vi "SetWaveLineColor.vi"(10 "曲线条数":u8, 11 "WaveformGraph输入":refnum<vi>) -> ()   [LabVIEW 2012, in "WaveGraphX.xctl"]
uses:
  WaveGraphX.xctl
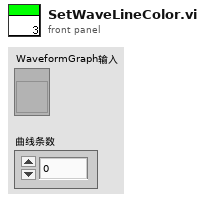
[diagram p1: front panel]
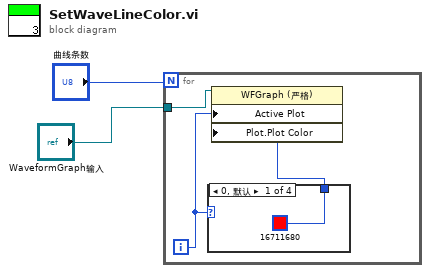
[diagram p0: block diagram]
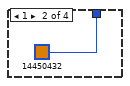
[diagram p2: hidden frame]
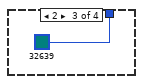
[diagram p3: hidden frame]
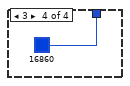
[diagram p4: hidden frame]
diagram:
  n1 = for {
    N: "曲线条数" -> [_]
    tunnel: "WaveformGraph输入" -> [w5]
    i -> [w4]
    n2 = case shown="0, 默认" w4 {
      tunnel: [u32 16711680 ("plot color") u32 14450432 ("plot color 2") u32 32639 ("plot color 3") u32 16860 ("plot color 4")] -> w3
      frame 0, Default {
      }
      frame 1 {
      }
      frame 2 {
      }
      frame 3 {
      }
    }
    n3 = property class="WFGraph (严格)"(reference=w5, "Active Plot"=w4, "Plot.Plot Color"=w3) -> ()  [unwired: 1 in, 2 out]
  }
